vi "Error - Log Error.vi"(8 "error in (no error)":errorcluster, 11 "Error Data":T1) -> (0 "error out":errorcluster)   [LabVIEW 2017]
doc: "Store all required Error data to external log file."
uses:
  Controls/Error Data.ctl
  Controls/Error Type.ctl
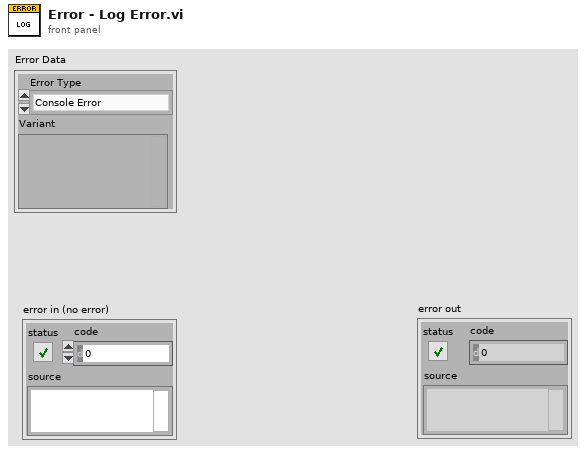
[diagram p1: front panel]
types:
  T1 = typedef "Error Data.ctl" = cluster{"Error Type":T2, "Variant":variant}
  T2 = typedef "Error Type.ctl" = enum16{"Console Error", "Sensor Interface IO Error", "Process Step Error"}
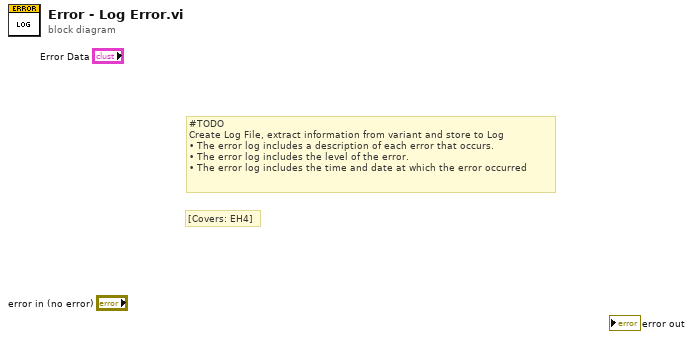
[diagram p0: block diagram]
diagram:
  # "[Covers: EH4]"
  # "#TODO\nCreate Log File, extract information from variant and store to Log\n• The error log includes a description of each error that occurs.\n• The error log includes the level of the error.\n• The error log includes the time and date at which the error occurred"
